vi "Read.vi"(8 "error in (no error)":errorcluster, 11 "Variant in":refnum<class "Variant.lvclass">) -> (0 "error out":errorcluster, 2 "Variant":variant, 3 "Variant out":refnum<class "Variant.lvclass">)   [LabVIEW 2020, in "Data.lvlib" / "Variant.lvclass"]
doc: "Read Variant."
uses:
  Variant.lvclass
  Variant.lvclass/Variant.ctl
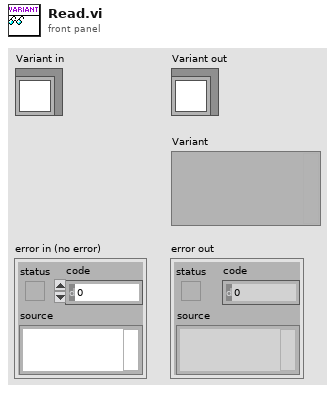
[diagram p1: front panel]
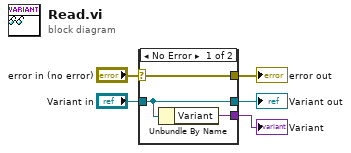
[diagram p0: block diagram]
diagram:
  n1 = case shown="No Error" "error in (no error)" {
    selector: "error in (no error)" -> [w8 w9]
    tunnel: [w8 w9] -> w4
    tunnel: [w7 w10] -> w2
    tunnel: "Variant in" -> [w7 w10]
    tunnel: [w6 _] -> w1
    frame No Error {
      n2 = Unbundle By Name(w7) -> ("Variant"=w6:variant)
    }
    frame Error {
    }
  }
  "error out" <- w4
  "Variant out" <- w2
  "Variant" <- w1
